vi "DB Tools Select All Data.vi"(4 "optional clause":string, 5 "error in (no error)":errorcluster, 6 "columns":string[](array[string]), 7 "table":string, 8 "connection reference":T1) -> (0 "error out":errorcluster, 1 "data":string[][](table), 3 "connection reference out":T1)   [LabVIEW 2012, in "NI_Database_API_64.lvlib"]
doc: "Selects data from the <B>table</B> in the database identified by <B>connection reference</B> using the columns supplied in the <B>columns</B> array. This VI uses the DB Tools Fetch Table Data to return the recordset into a 2D array of strings ( also a table data type in LabVIEW)."
uses:
  NI_Database_API_64.lvlib
  Connection.llb/Conn Execute.vi
  Recordset.llb/Rec Destroy - Connection.vi
  Connection.llb/Conn ObjectReference.ctl
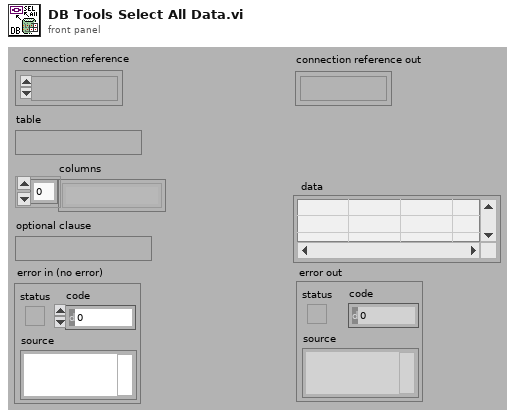
[diagram p1: front panel]
types:
  T1 = typedef "NI_Database_API_64.lvlib/Conn ObjectReference.ctl" = refnum<k1>
  T2 = typedef "NI_Database_API_64.lvlib/Rec ObjectReference.ctl" = refnum<k1>
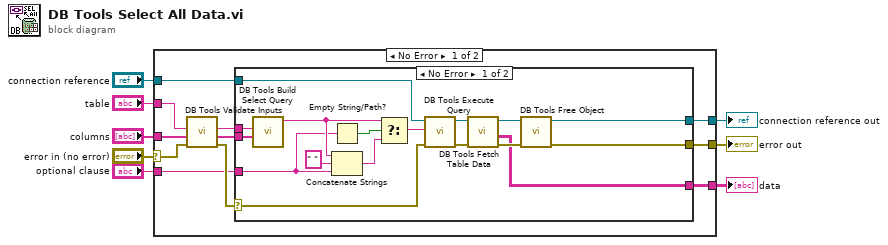
[diagram p0: block diagram]
diagram:
  n1 = case shown="No Error" "error in (no error)" {
    selector: "error in (no error)" -> [w9 w40]
    tunnel: "table" -> [w19 _]
    tunnel: [w18 w40] -> w7
    tunnel: "columns" -> [w14 _]
    tunnel: [w13 _] -> w5
    tunnel: "optional clause" -> [w12 _]
    tunnel: [w11 w39] -> w3
    tunnel: "connection reference" -> [w10 w39]
    frame No Error {
      n2 = call "DB Tools Validate Inputs.vi"("error in (no error)"=w9, "columns"=w14, "table"=w19) -> ("error out"=w15:errorcluster, "columns out"=w17:string[], "table out"=w16:string)  [unwired: 2 in]
      n3 = case shown="No Error" w15 {
        selector: w15 -> [w34 w38]
        tunnel: w17 -> [w36 _]
        tunnel: w16 -> [w35 _]
        tunnel: [w33 w38] -> w18
        tunnel: [w23 _] -> w13
        tunnel: w12 -> [w22 _]
        tunnel: [w21 w37] -> w11
        tunnel: w10 -> [w20 w37]
        frame No Error {
          n4 = call "DB Tools Build Select Query.vi"("columns"=w36, "table name"=w35) -> ("select query"=w31:string)  [unwired: 5 in]
          n5 = Empty String/Path?(string/path=w22) -> (empty?=w32:bool)
          n6 = Concatenate Strings(w31, " " ("Substring"), w22) -> (w30:string)
          n7 = Select(t=w31, s=w32, f=w30) -> (s? t:f=w28:string)
          n8 = call-poly "DB Tools Execute Query.vi"("error in (no error)"=w34, "SQL query"=w28, "connection reference"=w20) -> ("error out"=w26:errorcluster, "recordset reference"=w27:T2)  [unwired: 5 in]
          n9 = call "DB Tools Fetch Table Data.vi"("error in (no error)"=w26, "recordset reference"=w27) -> ("error out"=w25:errorcluster, "recordset data"=w23:string[][], "recordset reference out"=w24:T2)  [unwired: 3 in]
          n10 = call-poly "DB Tools Free Object.vi"("error in (no error)"=w25, "recordset reference"=w24) -> ("error out"=w33:errorcluster, "connection reference"=w21:T1)  [unwired: 8 in]
        }
        frame Error {
        }
      }
    }
    frame Error {
    }
  }
  "error out" <- w7
  "data" <- w5
  "connection reference out" <- w3
